vi "CSM - Global Log Event.vi"(6 "Timeout In ms (5000ms)":i32=5000, 8 "Error In":errorcluster caption="error in (no error)") -> (0 "error out":errorcluster, 3 "Global Log Event":refnum<user-event>)   [LabVIEW 2017, in "Communicable State Machine.lvlib"]
doc: "Obtains the CSM global log user event refnum, used to retrieve global log user events from the global log queue.\n\n\n> [!NOTE] <b>CSM Global Log Functionality</b>\n>\n> The CSM Global Log functionality is used to view global log change events, serving scenarios such as debugging and monitoring.\n> The following is the information that can be logged:\n> - Module state modifications\n> - Inter-module message communication, including data returns\n> - Message completion records of asynchronous and synchronous messages, `AsyncMsg Complete` and `SyncMsg Complete`, which carry the response\n> - Module status publishing\n> - Module creation and destruction\n> - Module state registration and unregistration\n> - Error information handled by modules\n> - User-defined events\n>\n> Debugging tools are primarily developed based on the Global Log API. You can develop debugging tools according to your own needs.\n\n\n> [!NOTE] <b>CSM Global Log Acquisition Methods</b>\n>\n> CSM provides two methods for acquiring global logs: Queue and Event. The Queue processing method is recommended because the queue interface is more efficient and offers greater flexibility in selecting log processing schemes based on the number of accumulated logs in the queue.\n\n\n<b>Reference Examples</b>:\n- `4. Advance Examples\\Filter From Source(Event).vi`\n- `4. Advance Examples\\Filter From Subscriber(Event).vi`\n\n-- <b>Indicators</b> --\n- <b>CSM Global Log Event</b>: CSM global log user event refnum.\n- <b>Timeout In ms (5000ms)</b>: Timeout duration. The default is 5000 ms."
uses:
  Communicable State Machine.lvlib
  _Support/Typedef/_CSM_GlobalLog_MSG.ctl
  _Support/Typedef/_CSM_Response Source Message.ctl
  _Support/Typedef/_CSM_GlobalLog_MSG_TYPE.ctl
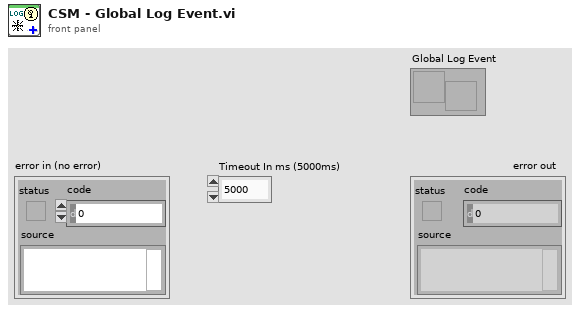
[diagram p1: front panel]
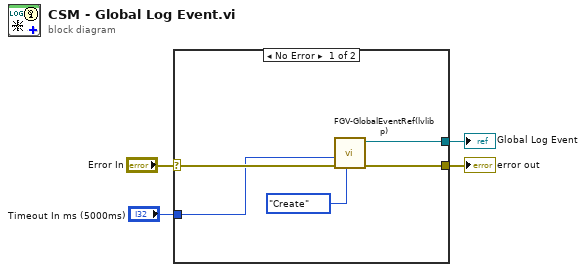
[diagram p0: block diagram]
diagram:
  n1 = case shown="No Error" "Error In" {
    selector: "Error In" -> [w8 w10]
    tunnel: [w9 w10] -> w4
    tunnel: [w7 _] -> w2
    tunnel: "Timeout In ms (5000ms)" -> [w6 _]
    frame No Error {
      n2 = call "FGV-GlobalEventRef(lvlibp).vi"("Operation"=enum16{"Create", "Read", "Destroy"}."Create", "error in (no error)"=w8, "Timeout In ms (5000 ms)"=w6) -> ("error out"=w9:errorcluster, "Event"=w7:refnum<user-event>)  [unwired: 7 in]
    }
    frame Error {
    }
  }
  "error out" <- w4
  "Global Log Event" <- w2
